vi "Add.vi"(8 "error in (no error)":errorcluster, 11 "Modulo a obtener":T1=enum."Error") -> (0 "error out":errorcluster)   [LabVIEW 2020]
uses:
  Comunes/Controles/Lista Modulos.ctl
  Comunes/Controles/Tallas.ctl
  Comunes/Controles/FGV Opciones.ctl
  Comunes/Comunicacion/Mensajes.lvlib
panel:
  in  "Color":string(combo)
  in  "Modelo":string(combo)
  in  "Talla":T2
  in  "Agregar zapato":bool
  in  "Color":string
  in  "Modelo":string
  in  "BtnNuevo color":bool
  in  "BtnNuevo Modelo":bool
  in  "BtnBorrarColor":bool caption="BtnNuevo color"
  in  "BtnBorrarModelo":bool caption="BtnNuevo color"
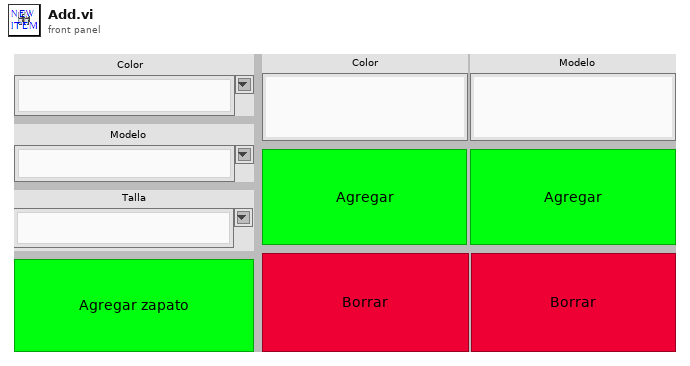
[diagram p1: front panel]
types:
  T1 = typedef "Lista Modulos.ctl" = enum16{"Math", "Error", "Front", "Database", "Nuevos items"}
  T2 = typedef "Tallas.ctl" = string
  T3 = typedef "FGV Opciones.ctl" = enum16{"Get", "Create", "Destroy"}
  T4 = enum32{"Invalid", "Standard", "Closed", "Hidden", "Minimized", "Maximized"}
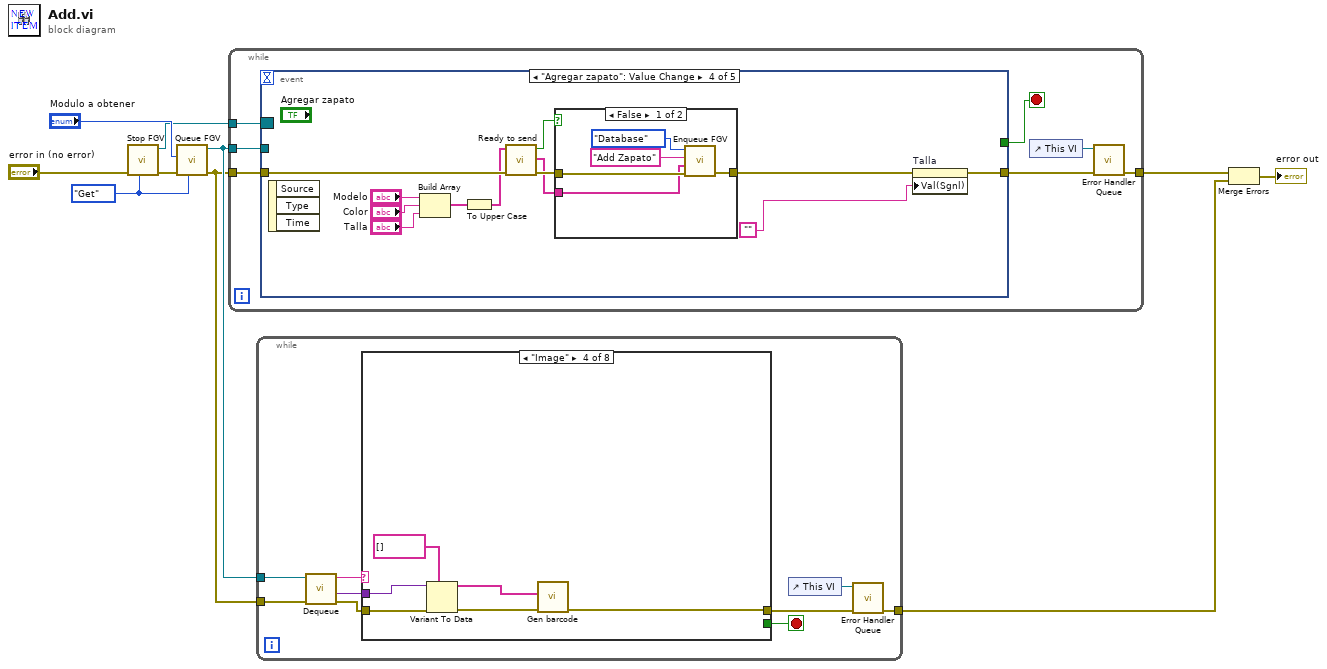
[diagram p0: block diagram]
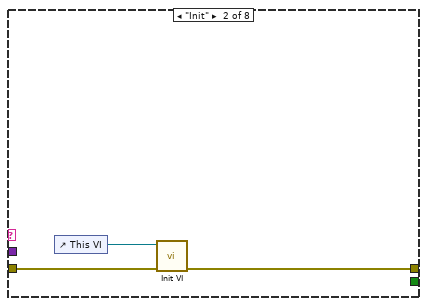
[diagram p3: hidden frame]
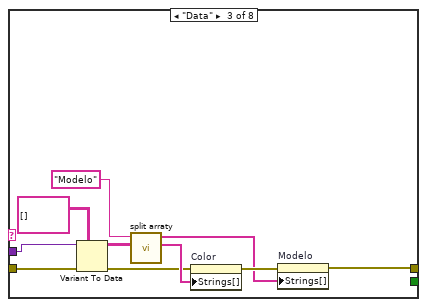
[diagram p4: hidden frame]
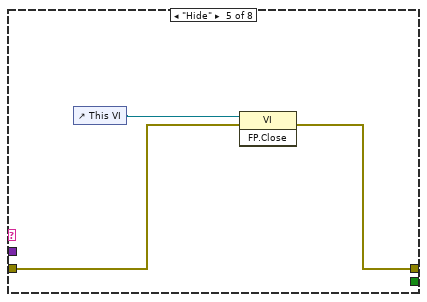
[diagram p5: hidden frame]
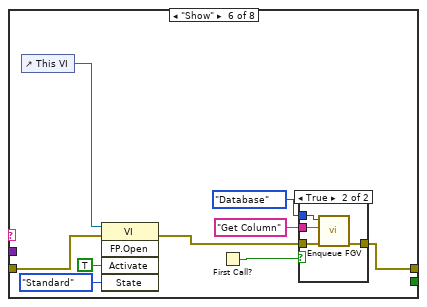
[diagram p6: hidden frame]
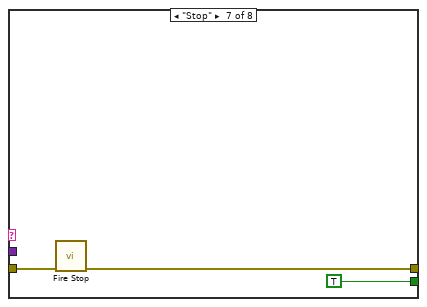
[diagram p8: hidden frame]
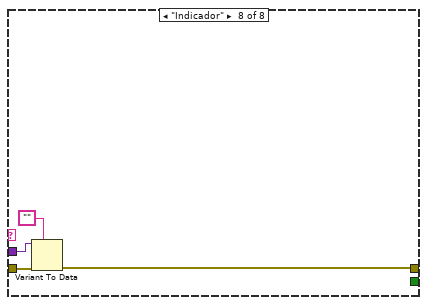
[diagram p9: hidden frame]
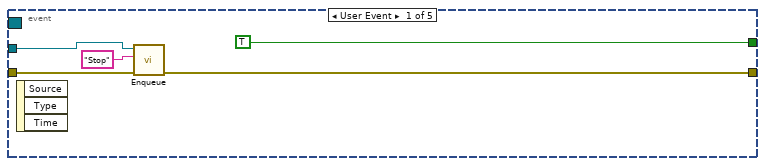
[diagram p10: hidden frame]
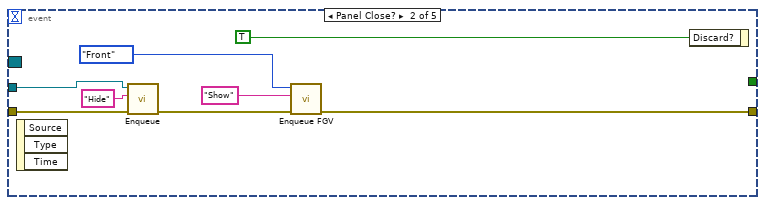
[diagram p11: hidden frame]
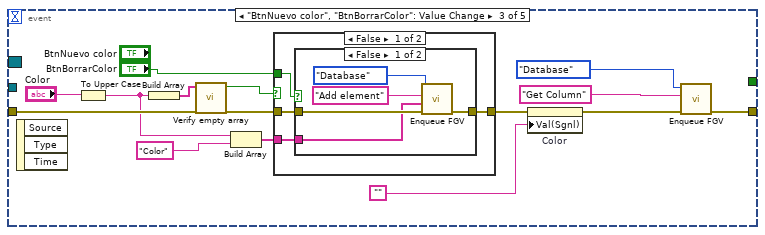
[diagram p12: hidden frame]
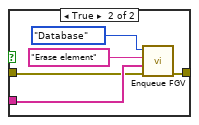
[diagram p13: hidden frame]
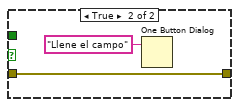
[diagram p14: hidden frame]
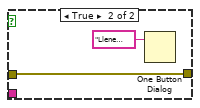
[diagram p15: hidden frame]
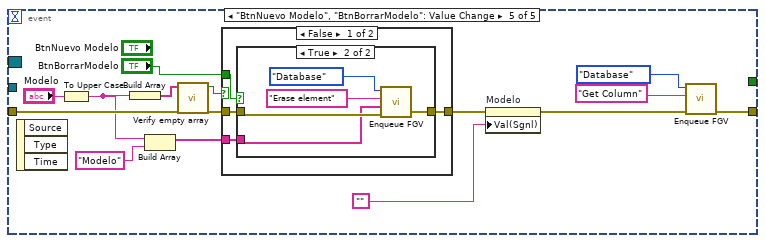
[diagram p16: hidden frame]
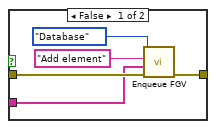
[diagram p17: hidden frame]
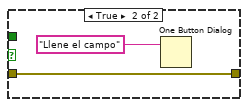
[diagram p18: hidden frame]
diagram:
  w1 = FGV_Opciones."Get" ("Enum")
  n1 = call "Stop FGV.vi"("Enum"=w1, "error in (no error)"="error in (no error)") -> ("error out"=w2:errorcluster, "Event Registration Refnum"=w4:refnum<event-registration>)  [unwired: 7 in, 1 out]
  n2 = call "Queue FGV.vi"("Enum"=w1, "error in (no error)"=w2, "Modulo a obtener"="Modulo a obtener") -> ("error out"=w8:errorcluster, "Queue Ref"=w9:refnum<queue>)  [unwired: 7 in]
  n3 = while {
    tunnel: w9 -> [w17]
    tunnel: w8 -> [w16]
    tunnel: [w14] -> w7
    tunnel: w4 -> [w12]
    stop <- w11 stop-if-true
    n4 = event shown="[3] \"Agregar zapato\": Value Change" {
      selector: w12 -> [_ _ _ _ _]
      dyn-events: _ -> [_ _ _ _ _]
      timeout: _ -> [_ _ _ _ _]
      tunnel: w17 -> [w20 w29 _ _ _]
      tunnel: w16 -> [w21 w28 w44 w68 w91]
      tunnel: [w18 w23 w35 w63 w84] -> w13
      tunnel: [TRUE _ _ _ _] -> w11
      event User Event {
        n5 = event-data() -> ()  [unwired: 1 in, 3 out]
        n6 = call "Enqueue.vi"("error in (no error)"=w21, "Mensaje"="Stop", "Queue in"=w20) -> ("error out"=w18:errorcluster)  [unwired: 8 in]
      }
      event Panel Close? {
        n7 = event-data() -> ()  [unwired: 1 in, 3 out]
        n8 = call "Enqueue.vi"("error in (no error)"=w28, "Mensaje"="Hide", "Queue in"=w29) -> ("error out"=w26:errorcluster)  [unwired: 8 in]
        n9 = call "Enqueue FGV.vi"("error in (no error)"=w26, "Mensaje"="Show", "Modulo a obtener"=Lista_Modulos."Front") -> ("error out"=w23:errorcluster)  [unwired: 8 in]
        n10 = event-data("Discard?"=TRUE) -> ()  [unwired: 1 in, 1 out]
      }
      event "BtnNuevo color", "BtnBorrarColor": Value Change {
        n11 = event-data() -> ()  [unwired: 1 in, 3 out]
        n12 = To Upper Case(1:"Color") -> (0:w32:string)
        n13 = Build Array(w32) -> (w43:string[])
        n14 = call "Verify empty array.vi"("Entradas"=w43) -> ("Is Null?"=w42:bool)  [unwired: 10 in]
        n15 = Build Array(w32, "Color" ("element")) -> (w39:string[])
        n16 = case shown="False" w42 {
          tunnel: [w48 w60] -> w41
          tunnel: w44 -> [w47 w60]
          tunnel: w39 -> [w46 _]
          tunnel: "BtnBorrarColor" -> [w45 _]
          frame False {
            n17 = case shown="False" w45 {
              tunnel: [w53 w54] -> w48
              tunnel: w47 -> [w52 w55]
              tunnel: w46 -> [w51 w56]
              frame False {
                n18 = call "Enqueue FGV.vi"("error in (no error)"=w52, "Dato"=w51, "Mensaje"="Add element", "Modulo a obtener"=Lista_Modulos."Database") -> ("error out"=w53:errorcluster)  [unwired: 7 in]
              }
              frame True {
                n19 = call "Enqueue FGV.vi"("error in (no error)"=w55, "Dato"=w56, "Mensaje"="Erase element", "Modulo a obtener"=Lista_Modulos."Database") -> ("error out"=w54:errorcluster)  [unwired: 7 in]
              }
            }
          }
          frame True {
            n20 = One Button Dialog(message="Llene el campo") -> ()  [unwired: 1 in, 1 out]
          }
        }
        n21 = property on="Color" class="Str"(error in=w41, "Val(Sgnl)"="") -> (error out=w34:errorcluster)  [unwired: 1 in, 1 out]
        n22 = call "Enqueue FGV.vi"("error in (no error)"=w34, "Mensaje"="Get Column", "Modulo a obtener"=Lista_Modulos."Database") -> ("error out"=w35:errorcluster)  [unwired: 8 in]
      }
      event "Agregar zapato": Value Change {
        n23 = event-data() -> ()  [unwired: 1 in, 3 out]
        n24 = Build Array("Modelo", "Color", "Talla") -> (w65:T2[])
        n25 = To Upper Case(1:w65) -> (0:w64:T2[])
        n26 = call "Ready to send.vi"("error in (no error)"=w68, "Entradas"=w64) -> ("error IO"=w69:errorcluster, "Resultante"=w66:string[], "Is Null?"=w67:bool)  [unwired: 6 in, 1 out]
        n27 = case shown="False" w67 {
          tunnel: [w77 w79] -> w61
          tunnel: w69 -> [w76 w79]
          tunnel: w66 -> [w73 _]
          frame False {
            n28 = call "Enqueue FGV.vi"("error in (no error)"=w76, "Dato"=w73, "Mensaje"="Add Zapato", "Modulo a obtener"=Lista_Modulos."Database") -> ("error out"=w77:errorcluster)  [unwired: 7 in]
          }
          frame True {
            n29 = One Button Dialog(message="Llene correctamente los campos") -> ()  [unwired: 1 in, 1 out]
          }
        }
        n30 = property on="Talla" class="CmbBox (strict)"(error in=w61, "Val(Sgnl)"="") -> (error out=w63:errorcluster)  [unwired: 1 in, 1 out]
      }
      event "BtnNuevo Modelo", "BtnBorrarModelo": Value Change {
        n31 = event-data() -> ()  [unwired: 1 in, 3 out]
        n32 = To Upper Case(1:"Modelo") -> (0:w81:string)
        n33 = Build Array(w81) -> (w93:string[])
        n34 = Build Array(w81, "Modelo" ("element")) -> (w88:string[])
        n35 = call "Verify empty array.vi"("Entradas"=w93) -> ("Is Null?"=w92:bool)  [unwired: 10 in]
        n36 = case shown="False" w92 {
          tunnel: [w97 w109] -> w90
          tunnel: w91 -> [w96 w109]
          tunnel: w88 -> [w95 _]
          tunnel: "BtnBorrarModelo" -> [w94 _]
          frame False {
            n37 = case shown="True" w94 {
              tunnel: [w102 w103] -> w97
              tunnel: w96 -> [w101 w105]
              tunnel: w95 -> [w100 w104]
              frame False {
                n38 = call "Enqueue FGV.vi"("error in (no error)"=w101, "Dato"=w100, "Mensaje"="Add element", "Modulo a obtener"=Lista_Modulos."Database") -> ("error out"=w102:errorcluster)  [unwired: 7 in]
              }
              frame True {
                n39 = call "Enqueue FGV.vi"("error in (no error)"=w105, "Dato"=w104, "Mensaje"="Erase element", "Modulo a obtener"=Lista_Modulos."Database") -> ("error out"=w103:errorcluster)  [unwired: 7 in]
              }
            }
          }
          frame True {
            n40 = One Button Dialog(message="Llene el campo") -> ()  [unwired: 1 in, 1 out]
          }
        }
        n41 = property on="Modelo" class="Str"(error in=w90, "Val(Sgnl)"="") -> (error out=w83:errorcluster)  [unwired: 1 in, 1 out]
        n42 = call "Enqueue FGV.vi"("error in (no error)"=w83, "Mensaje"="Get Column", "Modulo a obtener"=Lista_Modulos."Database") -> ("error out"=w84:errorcluster)  [unwired: 8 in]
      }
    }
    n43 = control-ref of="This VI"() -> (w15:refnum<vi>)
    n44 = call "Error Handler Queue.vi"("error in (no error)"=w13, "VI Refnum"=w15) -> ("error out"=w14:errorcluster)  [unwired: 9 in]
  }
  n45 = while {
    tunnel: w9 -> [w118]
    tunnel: w8 -> [w117]
    tunnel: [w111] -> w6
    stop <- w110 stop-if-true
    n46 = call "Dequeue.vi"("error in (no error)"=w117, "Queue in"=w118) -> ("error out"=w113:errorcluster, "Dato"=w115:variant, "Mensaje"=w116:string)  [unwired: 7 in]
    n47 = case shown="\"Image\"" w116 {
      tunnel: w115 -> [_ _ w131 w137 _ _ _ w161]
      tunnel: w113 -> [w119 w122 w132 w138 w140 w147 w158 w162]
      tunnel: [w119 w121 w123 w134 w139 w146 w156 w159] -> w112
      tunnel: [_ _ _ _ _ _ TRUE _] -> w110
      frame "False", Default {
      }
      frame "Init" {
        n48 = control-ref of="This VI"() -> (w120:refnum<vi>)
        n49 = call "Init VI.vi"("error in (no error)"=w122, "VI in"=w120) -> ("error out"=w121:errorcluster)  [unwired: 9 in]
      }
      frame "Data" {
        n50 = Variant To Data(error in=w132, type=string[][] [], Variant=w131) -> (data=w129:string[][], error out=w125:errorcluster)
        n51 = call "split arraty.vi"("Datos bruto"=w129, "Parametro"="Modelo") -> ("Datos segundo parametro"=w126:string[], "Datos parametro"=w124:string[])  [unwired: 8 in]
        n52 = property on="Color" class="CmbBox"(error in=w125, "Strings[]"=w126) -> (error out=w127:errorcluster)  [unwired: 1 in, 1 out]
        n53 = property on="Modelo" class="CmbBox"(error in=w127, "Strings[]"=w124) -> (error out=w123:errorcluster)  [unwired: 1 in, 1 out]
      }
      frame "Image" {
        n54 = Variant To Data(error in=w138, type=string[] [], Variant=w137) -> (data=w133:string[], error out=w135:errorcluster)
        n55 = call "Gen barcode.vi"("error in (no error)"=w135, "Full data"=w133) -> ("error out"=w134:errorcluster)  [unwired: 9 in]
      }
      frame "Hide" {
        n56 = control-ref of="This VI"() -> (w141:refnum<vi>)
        n57 = invoke class="VI" method="FP.Close"(reference=w141, error in=w140) -> (error out=w139:errorcluster)  [unwired: 1 in, 2 out]
      }
      frame "Show" {
        n58 = control-ref of="This VI"() -> (w148:refnum<vi>)
        n59 = invoke class="VI" method="FP.Open"(reference=w148, error in=w147, "Activate"=TRUE ("Activate?"), "State"=T4."Standard") -> (error out=w145:errorcluster)  [unwired: 1 in, 4 out]
        n60 = First Call?() -> (First Call?: T/F=w142:bool)
        n61 = case shown="True" w142 {
          tunnel: [w151 w155] -> w146
          tunnel: w145 -> [w151 w154]
          tunnel: Lista_Modulos."Database" ("Modulo a obtener") -> [_ w153]
          tunnel: "Get Column" ("Mensaje") -> [_ w152]
          frame False {
          }
          frame True {
            n62 = call "Enqueue FGV.vi"("error in (no error)"=w154, "Mensaje"=w152, "Modulo a obtener"=w153) -> ("error out"=w155:errorcluster)  [unwired: 8 in]
          }
        }
      }
      frame "Stop" {
        n63 = call "Fire Stop.vi"("error in (no error)"=w158) -> ("error out"=w156:errorcluster)  [unwired: 10 in]
      }
      frame "Indicador" {
        n64 = Variant To Data(error in=w162, type="", Variant=w161) -> (error out=w159:errorcluster)  [unwired: 1 out]
      }
    }
    n65 = control-ref of="This VI"() -> (w114:refnum<vi>)
    n66 = call "Error Handler Queue.vi"("error in (no error)"=w112, "VI Refnum"=w114) -> ("error out"=w111:errorcluster)  [unwired: 9 in]
  }
  n67 = Merge Errors(w7, w6) -> (→"error out":errorcluster)
